vi "Get Variant as String.vi"(9 "time format string (%c)":string, 10 "Digits of Precision":i16, 11 "Variant":variant) -> (3 "Variant Value as String":string)   [LabVIEW 2022 SP3, in "CSV Export.lvlib" / "CSV Export.lvclass"]
uses:
  CSV Export.lvclass
  <vilib>/Utility/Data Type/NI_Data Type.lvlib
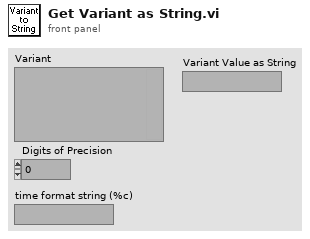
[diagram p1: front panel]
types:
  T1 = typedef "NI_Data Type.lvlib/Data Type.ctl" = enum8{"Invalid Type", "Void", "I8", "I16", "I32", "I64", "U8", "U16", "U32", "U64", "Single Float", "Double Float", "Extended Float", "Single Complex", "Double Complex", "Extended Complex", "Enum U8", "Enum U16", "Enum U32", "Enum U64", "Single Float With Unit", "Double Float With Unit", "Extended Float With Unit", "Single Complex with Unit", "Double Complex with Unit", "Extended Complex with Unit", "Boolean", "String", "Path", "Picture", "Tag", "Array", "Cluster", "Variant", "LV Variant", "Waveform", "Timestamp", "Digital Waveform", "Digital Data", "ExpressData", "Refnum", "External Data", "VI", "Poly VI", "LabVIEW Class Instance", "Fixed Point", "Set Collection", "Map Collection"}
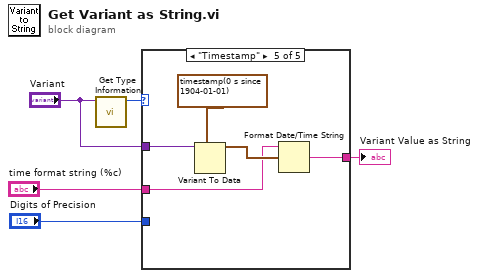
[diagram p0: block diagram]
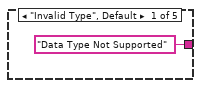
[diagram p2: hidden frame]
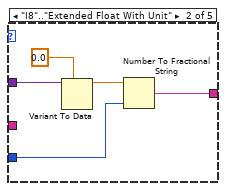
[diagram p3: hidden frame]
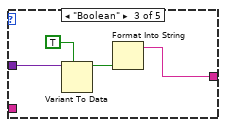
[diagram p4: hidden frame]
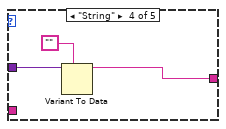
[diagram p5: hidden frame]
diagram:
  n1 = call <vilib>:"Get Type Information.vi"("variant"="Variant") -> ("type"=w5:T1)  [unwired: 6 in, 4 out]
  n2 = case shown="\"Timestamp\"" w5 {
    tunnel: "Variant" -> [_ w10 w15 w18 w23]
    tunnel: ["Data Type Not Supported" w8 w12 w16 w20] -> w1
    tunnel: "Digits of Precision" -> [_ w7 _ _ _]
    tunnel: "time format string (%c)" -> [_ _ _ _ w19]
    frame "Invalid Type", Default {
    }
    frame "I8".."Extended Float With Unit" {
      n3 = Variant To Data(type=0.0, Variant=w10) -> (data=w9:dbl)  [unwired: 1 in, 1 out]
      n4 = Number To Fractional String(number=w9, precision (6)=w7) -> (F-format string=w8:string)  [unwired: 2 in]
    }
    frame "Boolean" {
      n5 = Variant To Data(type=TRUE, Variant=w15) -> (data=w13:bool)  [unwired: 1 in, 1 out]
      n6 = Format Into String(w13) -> (resulting string=w12:string)  [unwired: 3 in, 1 out]
    }
    frame "String" {
      n7 = Variant To Data(type="", Variant=w18) -> (data=w16:string)  [unwired: 1 in, 1 out]
    }
    frame "Timestamp" {
      n8 = Variant To Data(type=timestamp(0 s since 1904-01-01) ("time stamp"), Variant=w23) -> (data=w21:timestamp)  [unwired: 1 in, 1 out]
      n9 = Format Date/Time String(time format string (%c)=w19, seconds (now)=w21) -> (date/time string=w20:string)  [unwired: 1 in]
    }
  }
  "Variant Value as String" <- w1
